vi "PS-OCTA-OCE-autofocus.vi"() -> ()   [LabVIEW 2024] (continued)
                                n349 = call "ORS_Fit_Recalibration_Fringes_Jay.vi"("polynomial order"="poly order", "n Recalibration Fringes"=w812, "polynomial fit algorithm"=T11."LU Decomposition" ("poly fit algo"), "moving average half width"="moving avg win", "interpolation method"=w828, "doPolyFit"="doPolyFit", "Offset"=w791, "Length"=w790) -> ("maxphase"=w795:dbl, "phase"=w797:dbl[], "inverted phase"=w804:dbl[], "rel.phase error"=w807:dbl[])  [unwired: 4 in]
                                n350 = for {
                                tunnel: w823 -> [w839] mode=indexing
                                tunnel: [w838] -> w811 mode=indexing
                                n351 = call-poly <vilib>:"Mean.vi"("X"=w839) -> ("mean"=w838:dbl)  [unwired: 1 out]
                                }
                                n352 = disable-structure shown="Disabled" {
                                disable-tunnel: w807 -> [w831 _]
                                frame Disabled {
                                "Debug: Rel. phase error" <- w831
                                }
                                frame Enabled {
                                }
                                }
                                n353 = Array Size(array=w797) -> (size(s)=w799:i32)
                                n354 = call-poly <vilib>:"Ramp Pattern.vi"("start"=0.0, "end"=1.0, "samples"=w799) -> ("Ramp Pattern"=w796:dbl[])  [unwired: 7 in, 1 out]
                                n355 = call "ORS_linearize_Hilbert.vi"("# zeros added"="# zeros added", "Ch1 Michelson"=w811, "Hilbert in"=w797, "interpolation method"=w824) -> ("Ch1 linearized"=w822:dbl[])  [unwired: 6 in, 1 out]
                                n356 = case shown="True" "DoInterp" {
                                tunnel: w797 -> [_ w837]
                                tunnel: [w832 w837] -> w806
                                tunnel: [w832 w833] -> w805
                                tunnel: w804 -> [_ w834]
                                tunnel: w796 -> [w832 _]
                                frame False {
                                }
                                frame True {
                                n357 = In Range and Coerce(upper limit=1.0, x=w834, lower limit=0.0) -> (coerced(x)=w833:dbl[])  [unwired: 1 out]
                                }
                                }
                                n358 = Bundle By Name("Y"=w822, "dt"=w821) -> (w820:waveform(dbl))  [unwired: 1 in]
                                n359 = call-poly <vilib>:"Extract Single Tone Information.vi"("time signal in"=w820) -> ("detected frequency"=→"detected frequency":dbl)  [unwired: 5 in, 5 out]
                                n360 = Build Array(w806, w805) -> (w802:dbl[][])
                                n361 = Transpose 2D Array(2D array=w802) -> (transposed array=w801:dbl[][])
                              }
                              n362 = case shown="False" "DualCali" {
                                tunnel: w676 -> [w688 w760]
                                tunnel: w674 -> [w687 w759]
                                tunnel: w668 -> [w686 w758]
                                tunnel: w666 -> [w685 w757]
                                tunnel: w665 -> [w684 w756]
                                tunnel: w664 -> [w683 w755]
                                tunnel: [w682 w754] -> w663
                                tunnel: [w679 w753] -> w660
                                tunnel: w661 -> [w679 w753]
                                tunnel: "2ndCali" -> [w681 _]
                                tunnel: w658 -> [w680 _]
                                tunnel: w657 -> [w678 _]
                                frame True {
                                n363 = case shown="True" w686 {
                                tunnel: w688 -> [_ w698]
                                tunnel: [w689 w697] -> w682
                                tunnel: w687 -> [_ w696]
                                tunnel: w685 -> [w689 w694]
                                tunnel: w683 -> [_ w693]
                                tunnel: w684 -> [_ w695]
                                tunnel: w681 -> [_ w692]
                                tunnel: w680 -> [_ w691]
                                tunnel: w678 -> [_ w690]
                                frame False {
                                }
                                frame True {
                                n364 = case shown="True" w692 {
                                tunnel: w698 -> [w701 w710]
                                tunnel: [w702 w709] -> w697
                                tunnel: w696 -> [_ w708]
                                tunnel: w695 -> [_ w707]
                                tunnel: w694 -> [w702 w706]
                                tunnel: w693 -> [_ w705]
                                tunnel: w691 -> [_ w704]
                                tunnel: w690 -> [w699 w703]
                                frame False {
                                n365 = Multiply(x=w701, y=w699) -> (x*y=→"caliphase":dbl[][])
                                }
                                frame True {
                                n366 = stacked-sequence {
                                seq-local: [w713 _] -> [_ w724]
                                tunnel: w710 -> [w722 w730]
                                tunnel: [_ w729] -> w709
                                tunnel: w708 -> [_ w728]
                                tunnel: w707 -> [_ w727]
                                tunnel: w706 -> [_ w726]
                                tunnel: w705 -> [_ w725]
                                tunnel: w704 -> [w712 _]
                                tunnel: w703 -> [w720 _]
                                frame #0 {
                                w717 = 0 ("index (row)")
                                n367 = Multiply(x=w722, y=w720) -> (x*y=w721:dbl[][])
                                n368 = local read "caliphase"() -> (w723:dbl[][])
                                n369 = Subtract(x=w721, y=w723) -> (x-y=w715:dbl[][])
                                n370 = Absolute Value(x=w715) -> (abs(x)=w714:dbl[][])
                                n371 = Index Array(array=w714, index (row)=w717, index (col)=w717) -> (element=w718:dbl)
                                n372 = Subtract(x=w714, y=w718) -> (x-y=w716:dbl[][])
                                n373 = Array Max & Min(array=w716) -> (max value=w719:dbl)  [unwired: 3 out]
                                n374 = Divide(x=w716, y=w719) -> (x/y=w713:dbl[][])
                                n375 = Subtract(x=w713, y=w712) -> (x-y=→"phasedif":dbl[][])
                                }
                                frame #1 {
                                n376 = case shown="False" w727 {
                                tunnel: w730 -> [_ _]
                                tunnel: [w732 w749] -> w729
                                tunnel: w728 -> [w736 w752]
                                tunnel: w726 -> [w734 w748]
                                tunnel: w725 -> [w733 w750]
                                tunnel: w724 -> [w731 w746]
                                frame True {
                                n377 = for {
                                N: 2 -> [_]
                                tunnel: w731 -> [w737]
                                tunnel: w736 -> [w745]
                                tunnel: w733 -> [w743]
                                shift-right: [w741] -> w732
                                shift-left: w734 -> [w740]
                                i -> [w744]
                                n378 = Subtract(x=w743, y=w744) -> (x-y=w738:i32)
                                n379 = Index Array(array=w740, index=w738) -> (element=w742:T13)
                                n380 = Bundle By Name(cluster=w742, "RecalFringePhaseFit"=w737, "RawRecalFringeArray"=w745) -> (w739:T13)
                                n381 = Replace Array Subset(array=w740, new element=w739, index=w738) -> (w741:T8)
                                }
                                }
                                frame False {
                                n382 = Index Array(array=w748, index=w750) -> (element=w751:T13)
                                n383 = Bundle By Name(cluster=w751, "RecalFringePhaseFit"=w746, "RawRecalFringeArray"=w752) -> (w747:T13)
                                n384 = Replace Array Subset(array=w748, new element=w747, index=w750) -> (w749:T8)
                                }
                                }
                                }
                                }
                                }
                                }
                                }
                                }
                                }
                                frame False {
                                n385 = case shown="True" w758 {
                                tunnel: w760 -> [_ w767]
                                tunnel: [w761 w766] -> w754
                                tunnel: w759 -> [_ w765]
                                tunnel: w757 -> [w761 w763]
                                tunnel: w755 -> [_ w762]
                                tunnel: w756 -> [_ w764]
                                frame False {
                                }
                                frame True {
                                n386 = case shown="False" w764 {
                                tunnel: w767 -> [w773 w789]
                                tunnel: [w768 w785] -> w766
                                tunnel: w765 -> [w772 w788]
                                tunnel: w763 -> [w770 w784]
                                tunnel: w762 -> [w769 w786]
                                frame True {
                                n387 = for {
                                N: 2 -> [_]
                                tunnel: w773 -> [w782]
                                tunnel: w772 -> [w781]
                                tunnel: w769 -> [w779]
                                shift-right: [w777] -> w768
                                shift-left: w770 -> [w776]
                                i -> [w780]
                                n388 = Subtract(x=w779, y=w780) -> (x-y=w774:i32)
                                n389 = Index Array(array=w776, index=w774) -> (element=w778:T13)
                                n390 = Bundle By Name(cluster=w778, "RecalFringePhaseFit"=w782, "RawRecalFringeArray"=w781) -> (w775:T13)
                                n391 = Replace Array Subset(array=w776, new element=w775, index=w774) -> (w777:T8)
                                }
                                }
                                frame False {
                                n392 = Index Array(array=w784, index=w786) -> (element=w787:T13)
                                n393 = Bundle By Name(cluster=w787, "RecalFringePhaseFit"=w789, "RawRecalFringeArray"=w788) -> (w783:T13)
                                n394 = Replace Array Subset(array=w784, new element=w783, index=w786) -> (w785:T8)
                                }
                                }
                                }
                                }
                                }
                              }
                            }
                            n395 = Transpose 2D Array(2D array=w651) -> (transposed array=→"Debug: Final phase fit":dbl[][])
                            n396 = Bundle By Name(cluster=w653, "Per Channel Params"=w648) -> (w655:T7)
                          }
                        }
                      }
                      frame #2 {
                        n397 = case shown="\"RecalFringe\", \"RecalFringesMirror\"" w864 {
                          frame "False", Default {
                          }
                          frame "RecalFringe", "RecalFringesMirror" {
                            n398 = Get Date/Time String(want seconds? (F)=TRUE ("Angabe von Sekunden? (F)")) -> (time string=→"Time of last RecalFringes":string)  [unwired: 2 in, 1 out]
                          }
                        }
                        n399 = local write "Acquire Recal Fringes with Mirror"(FALSE ("Capture background")) -> ()
                        n400 = local write "Apply Acq Config"(TRUE ("Apply Acq Config")) -> ()
                        n401 = Build Array (concatenate)(w866, "SaveState") -> (w867:string[])
                      }
                    }
                  }
                }
              }
            }
          }
          frame "Img:Preview" {
            # "Mode/ Tab selector"
            n402 = feedback #2() -> (w871:bool)  [unwired: 1 in]
            n403 = stacked-sequence {
              seq-local: [w913 _] -> [_ w1102]
              seq-local: [w897 _] -> [_ w1082]
              seq-local: [w903 _] -> [_ w1081]
              seq-local: [w912 _] -> [_ w1098]
              seq-local: [w911 _] -> [_ w1096]
              seq-local: [w910 _] -> [_ w1095]
              seq-local: [w909 _] -> [_ w1094]
              seq-local: [w908 _] -> [_ w1093]
              seq-local: [w907 _] -> [_ w1091]
              seq-local: [w906 _] -> [_ w1089]
              seq-local: [w905 _] -> [_ w1087]
              seq-local: [w904 _] -> [_ w1084]
              seq-local: [w896 _] -> [_ w1080]
              seq-local: [w945 _] -> [_ w1090]
              seq-local: [w917 _] -> [_ w1086]
              tunnel: w895 -> [w956 _]
              tunnel: w894 -> [w913 _]
              tunnel: w890 -> [w903 _]
              tunnel: w888 -> [w912 _]
              tunnel: w886 -> [w911 _]
              tunnel: w884 -> [w910 _]
              tunnel: w883 -> [w909 _]
              tunnel: w882 -> [w908 _]
              tunnel: w880 -> [w907 _]
              tunnel: w879 -> [w906 _]
              tunnel: w877 -> [w905 _]
              tunnel: w876 -> [w916 _]
              tunnel: w874 -> [w904 _]
              tunnel: w871 -> [_ _]
              tunnel: [_ w1101] -> w893
              tunnel: [_ w1082] -> w872
              tunnel: [_ w1100] -> w892
              tunnel: [_ w1081] -> w891
              tunnel: [_ w1099] -> w889
              tunnel: [_ w1097] -> w887
              tunnel: [_ w1085] -> w885
              tunnel: [_ w1092] -> w881
              tunnel: [_ w1088] -> w878
              tunnel: [_ w1086] -> w875
              tunnel: [_ w1083] -> w873
              frame #0 {
                # "Store all imaging parameters in the general state cluster"
                n404 = local read "Free running"() -> (w946:bool)
                n405 = Select(t=0, s=w946, f=-1) -> (s? t:f=w902:i32)
                n406 = Empty Array?(array=w916) -> (empty?=w915:bool)
                n407 = case shown="True" "show overlay?" {
                  tunnel: w916 -> [w1056 w1061]
                  tunnel: [w1057 w1063] -> w917
                  tunnel: w915 -> [w1058 w1062]
                  frame False {
                    n408 = case shown="False" w1058 {
                      tunnel: [u8[][] [] w1060] -> w1057
                      tunnel: w1056 -> [_ w1060]
                      frame False {
                      }
                      frame True {
                      }
                    }
                  }
                  frame True {
                    n409 = case shown="True" w1062 {
                      tunnel: [w1064 w1069] -> w1063
                      tunnel: w1061 -> [w1064 _]
                      frame False {
                      }
                      frame True {
                        n410 = Build Path(base path=path "states", name or relative path="overlay image name") -> (appended path=w1071:path)
                        n411 = call <vilib>:"Read PNG File.vi"("path to PNG file"=w1071) -> ("error out"=w1066:errorcluster, "image data"=w1070:T21)  [unwired: 8 in, 1 out]
                        n412 = Unbundle By Name(w1066) -> ("status"=w1068:bool)
                        n413 = call <vilib>:"Unflatten Pixmap.vi"("image data"=w1070) -> ("8-bit pixmap"=w1069:u8[][])  [unwired: 4 in, 6 out]
                        n414 = Not(x=w1068) -> (.not. x?=w1067:bool)
                        n415 = local write "show overlay?"(w1067) -> ()
                      }
                    }
                  }
                }
                n416 = event shown="[0] Timeout" {
                  selector: _ -> [_ _ _ _ _ _ _ _ _ _]
                  dyn-events: _ -> [_ _ _ _ _ _ _ _ _ _]
                  timeout: w902 -> [_ _ _ _ _ _ _ _ _ _]
                  tunnel: [_ _ _ TRUE _ _ _ _ _ _] -> w897
                  tunnel: ["DoPreview" "DoPreview" "DoPreview" "none" "none" "Scan3D" "DoPreview" "DoPreview" "DoPreview" "Do Preview"] -> w896
                  tunnel: "OCE_control" -> [_ _ _ _ _ _ _ w993 _ _]
                  tunnel: "OCT_control" -> [_ _ _ _ _ _ _ _ w1015 _]
                  tunnel: "OCTA_control" -> [_ _ _ _ _ _ w968 _ _ _]
                  tunnel: "Robot_control" -> [_ _ _ _ _ _ _ _ _ w1034]
                  event Timeout {
                    n417 = event-data() -> ()  [unwired: 1 in, 2 out]
                  }
                  event "3D preview": Value Change {
                    n418 = event-data() -> ()  [unwired: 1 in, 6 out]
                    n419 = local write "Apply Config"(TRUE ("Apply Config")) -> ()
                  }
                  event "Apply Acq param": Value Change {
                    n420 = event-data() -> ()  [unwired: 1 in, 6 out]
                    n421 = local write "Apply Config"(TRUE ("Apply Config")) -> ()
                  }
                  event "exit": Mouse Down; "exit": Key Down {
                    n422 = event-data() -> ()  [unwired: 1 in, 5 out]
                  }
                  event "OpModeTab": Value Change {
                    n423 = event-data() -> ()  [unwired: 1 in, 6 out]
                  }
                  event "Start 3D scan": Mouse Down; "Start 3D scan": Key Down; "trigger_scan": Value Change {
                    n424 = event-data() -> ()  [unwired: 1 in, 4 out]
                  }
                  event "OCTA_control": Value Change {
                    n425 = event-data() -> ()  [unwired: 1 in, 6 out]
                    n426 = local read "3D_Galvo_Params"() -> (w969:T4)
                    n427 = case shown="True" w968 {
                      tunnel: [w972 w988] -> w971
                      tunnel: w969 -> [w972 w989]
                      frame False {
                      }
                      frame True {
                        w973 = FALSE
                        n428 = local write "Apply Config"(TRUE) -> ()
                        n429 = local read "3D_Galvo_Params2_OCTA"() -> (w987:T4)
                        n430 = local write "OCT_control"(w973) -> ()
                        n431 = local write "Robot_control"(w973) -> ()
                        n432 = local write "OCE_control"(w973) -> ()
                        n433 = Unbundle By Name(w987) -> ("mode"=w986:i32, "n_lines"=w985:i32, "f_per_pos"=w984:i32, "n_frames"=w983:i32, "X center"=w982:dbl, "X span"=w981:dbl, "Y center"=w980:dbl, "Y span"=w979:dbl, "flyb.lines"=w978:i32, "galvo phase"=w977:i32, "n_dataset"=w976:u32, "flyback fr"=w975:u16)
                        n434 = Bundle By Name(cluster=w989, "mode"=w986, "n_lines"=w985, "f_per_pos"=w984, "n_frames"=w983, "X center"=w982, "X span"=w981, "Y center"=w980, "Y span"=w979, "flyb.lines"=w978, "galvo phase"=w977, "n_dataset"=w976, "flyback fr"=w975) -> (w988:T4)
                      }
                    }
                    n435 = local write "3D_Galvo_Params"(w971) -> ()
                  }
                  event "OCE_control": Value Change {
                    n436 = event-data() -> ()  [unwired: 1 in, 6 out]
                    n437 = local read "3D_Galvo_Params"() -> (w991:T4)
                    n438 = case shown="True" w993 {
                      tunnel: [w994 w1010] -> w992
                      tunnel: w991 -> [w994 w1011]
                      frame False {
                      }
                      frame True {
                        w995 = FALSE
                        n439 = local write "Apply Config"(TRUE) -> ()
                        n440 = local read "3D_Galvo_Params3_OCE"() -> (w997:T4)
                        n441 = local write "OCTA_control"(w995) -> ()
                        n442 = local write "OCT_control"(w995) -> ()
                        n443 = local write "Robot_control"(w995) -> ()
                        n444 = Unbundle By Name(w997) -> ("mode"=w1009:i32, "n_lines"=w1008:i32, "f_per_pos"=w1007:i32, "n_frames"=w1006:i32, "X center"=w1005:dbl, "X span"=w1004:dbl, "Y center"=w1003:dbl, "Y span"=w1002:dbl, "flyb.lines"=w1001:i32, "galvo phase"=w1000:i32, "n_dataset"=w999:u32, "flyback fr"=w998:u16)
                        n445 = Bundle By Name(cluster=w1011, "mode"=w1009, "n_lines"=w1008, "f_per_pos"=w1007, "n_frames"=w1006, "X center"=w1005, "X span"=w1004, "Y center"=w1003, "Y span"=w1002, "flyb.lines"=w1001, "galvo phase"=w1000, "n_dataset"=w999, "flyback fr"=w998) -> (w1010:T4)
                      }
                    }
                    n446 = local write "3D_Galvo_Params"(w992) -> ()
                  }
                  event "OCT_control": Value Change {
                    n447 = event-data() -> ()  [unwired: 1 in, 6 out]
                    n448 = local read "3D_Galvo_Params"() -> (w1014:T4)
                    n449 = case shown="True" w1015 {
                      tunnel: w1014 -> [w1016 w1022]
                      tunnel: [w1016 w1019] -> w1013
                      frame False {
                      }
                      frame True {
                        w1017 = FALSE
                        n450 = local write "Apply Config"(TRUE) -> ()
                        n451 = local read "3D_Galvo_Params4_OCT"() -> (w1021:T4)
                        n452 = local write "OCTA_control"(w1017) -> ()
                        n453 = local write "OCE_control"(w1017) -> ()
                        n454 = local write "Robot_control"(w1017) -> ()
                        n455 = Unbundle By Name(w1021) -> ("mode"=w1033:i32, "n_lines"=w1032:i32, "f_per_pos"=w1031:i32, "n_frames"=w1030:i32, "X center"=w1029:dbl, "X span"=w1028:dbl, "Y center"=w1027:dbl, "Y span"=w1026:dbl, "flyb.lines"=w1025:i32, "galvo phase"=w1024:i32, "n_dataset"=w1023:u32, "flyback fr"=w1020:u16)
                        n456 = Bundle By Name(cluster=w1022, "mode"=w1033, "n_lines"=w1032, "f_per_pos"=w1031, "n_frames"=w1030, "X center"=w1029, "X span"=w1028, "Y center"=w1027, "Y span"=w1026, "flyb.lines"=w1025, "galvo phase"=w1024, "n_dataset"=w1023, "flyback fr"=w1020) -> (w1019:T4)
                      }
                    }
                    n457 = local write "3D_Galvo_Params"(w1013) -> ()
                  }
                  event "Robot_control": Value Change {
                    n458 = event-data() -> ()  [unwired: 1 in, 6 out]
                    n459 = local read "3D_Galvo_Params"() -> (w1037:T4)
                    n460 = case shown="True" w1034 {
                      tunnel: w1037 -> [w1038 w1044]
                      tunnel: [w1038 w1041] -> w1036
                      frame False {
                      }
                      frame True {
                        w1039 = FALSE
                        n461 = local read "3D_Galvo_Params5_Robot"() -> (w1043:T4)
                        n462 = local write "Apply Config"(TRUE) -> ()
                        n463 = local write "OCTA_control"(w1039) -> ()
                        n464 = local write "OCE_control"(w1039) -> ()
                        n465 = local write "OCT_control"(w1039) -> ()
                        n466 = Unbundle By Name(w1043) -> ("mode"=w1055:i32, "n_lines"=w1054:i32, "f_per_pos"=w1053:i32, "n_frames"=w1052:i32, "X center"=w1051:dbl, "X span"=w1050:dbl, "Y center"=w1049:dbl, "Y span"=w1048:dbl, "flyb.lines"=w1047:i32, "galvo phase"=w1046:i32, "n_dataset"=w1045:u32, "flyback fr"=w1042:u16)
                        n467 = Bundle By Name(cluster=w1044, "mode"=w1055, "n_lines"=w1054, "f_per_pos"=w1053, "n_frames"=w1052, "X center"=w1051, "X span"=w1050, "Y center"=w1049, "Y span"=w1048, "flyb.lines"=w1047, "galvo phase"=w1046, "n_dataset"=w1045, "flyback fr"=w1042) -> (w1041:T4)
                      }
                    }
                    n468 = local write "3D_Galvo_Params"(w1036) -> ()
                  }
                }
                n469 = Unbundle By Name(w956) -> ("Per Channel Params"=w958:T8)
                n470 = local read "Dispersion coef"() -> (w943:dbl)
                n471 = local read "cut_level_low"() -> (w954:dbl)
                n472 = local read "cut_level_high"() -> (w953:dbl)
                n473 = local read "crop start"() -> (w955:i32)
                n474 = local read "DVV shift"() -> (w944:i32)
                n475 = for {
                  tunnel: w958 -> [w1079] mode=indexing
                  tunnel: [w1077] -> w957 mode=indexing
                  tunnel: w955 -> [w1078]
                  tunnel: w954 -> [w1076]
                  tunnel: w953 -> [w1075]
                  tunnel: w944 -> [w1074]
                  tunnel: w943 -> [w1073]
                  n476 = Bundle By Name(cluster=w1079, "image crop start"=w1078, "cut_level_low"=w1076, "cut_level_high"=w1075, "DVV_shift"=w1074, "disp_coef"=w1073) -> (w1077:T13)
                }
                n477 = local read "PhaseCompVector"() -> (w928:cdb[])
                n478 = local read "FFT Down Sample"() -> (w924:i32)
                n479 = local read "Dispersion coef"() -> (w927:dbl)
                n480 = local read "cut_level_high"() -> (w923:dbl)
                n481 = local read "IgnoreBadClk"() -> (w920:bool)
                n482 = local read "image height"() -> (w951:i32)
                n483 = local read "DoDispComp"() -> (w929:bool)
                n484 = local read "cut_level_low"() -> (w922:dbl)
                n485 = local read "3D_Galvo_Params"() -> (w949:T4)
                n486 = local read "B scan offset"() -> (w952:dbl)
                n487 = local read "Enable DVV?"() -> (w932:bool)
                n488 = local read "ChannelDisp"() -> (w926:i32)
                n489 = local read "Override Ch."() -> (w934:bool[])
                n490 = local read "Good_Clock"() -> (w919:dbl)
                n491 = local read "Description"() -> (w941:string)
                n492 = local read "Disable Bck"() -> (w930:bool[])
                n493 = local read "ATS_clock 2"() -> (w938:T1)
                n494 = local read "OCT NAME"() -> (w950:string)
                n495 = local read "OCT Zoom"() -> (w925:sgl)
                n496 = local read "Bad_Clock"() -> (w918:dbl)
                n497 = local read "OCT PATH"() -> (w942:path)
                n498 = local read "dual_card"() -> (w940:bool)
                n499 = local read "ATS_clock"() -> (w939:T1)
                n500 = local read "Ch. Select"() -> (w935:bool[])
                n501 = local read "DoInterp"() -> (w933:bool)
                n502 = local read "digi_trig"() -> (w936:bool)
                n503 = local read "Channel"() -> (w921:u32)
                n504 = local read "AO.type"() -> (w931:i32)
                n505 = local read "DES"() -> (w937:bool)
                n506 = Bundle By Name(cluster=w956, "Per Channel Params"=w957, "image height (crop)"=w951, "B scan offset (sps)"=w952, "OCT data dir"=w942, "3d file name"=w950, "Description"=w941, "Galvo params only for file storage"=w949, "do_dual_card"=w940, "ATS_clock"=w939, "ATS_clock 2"=w938, "DES"=w937, "digi_trig"=w936, "Ch. Select"=w935, "Override Ch."=w934, "DoInterp"=w933, "EnableDVV"=w932, "AO.type"=w931, "Disable Bck"=w930, "PhaseCompVector"=w928, "DoDispComp"=w929, "dispcoef"=w927, "ChannelDisp"=w926, "Zoom Factor"=w925, "FFT Down Sample"=w924, "cut_level_high"=w923, "cut_level_low"=w922, "Channel"=w921, "IgnoreBadClk"=w920, "Good_Clock"=w919, "Bad_Clock"=w918) -> (w945:T7)
              }
              frame #1 {
                n507 = case shown="\"DoPreview\"" w1080 {
                  tunnel: w1090 -> [w1175 w1494 w1994]
                  tunnel: w1102 -> [w1201 w1496 w1993]
                  tunnel: [w1175 w1493 w1994] -> w1101
                  tunnel: [w1197 w1495 w1993] -> w1100
                  tunnel: [w1200 _ _] -> w1099
                  tunnel: w1098 -> [w1169 _ _]
                  tunnel: [w1199 _ _] -> w1097
                  tunnel: w1096 -> [w1162 _ _]
                  tunnel: [w1172 _ _] -> w1085
                  tunnel: w1095 -> [w1173 _ _]
                  tunnel: w1094 -> [_ w1492 _]
                  tunnel: w1093 -> [_ w1491 _]
                  tunnel: [w1198 _ _] -> w1092
                  tunnel: w1091 -> [_ _ _]
                  tunnel: w1089 -> [_ _ _]
                  tunnel: [w1161 _ _] -> w1088
                  tunnel: w1087 -> [w1160 _ _]
                  tunnel: w1086 -> [w1184 _ _]
                  tunnel: w1084 -> [w1146 _ _]
                  tunnel: [w1145 _ _] -> w1083
                  frame "DoPreview" {
                    # "frame_width"
                    n508 = stacked-sequence {
                      seq-local: [w1340 _ _ _] -> [_ w1350 _ _]
                      seq-local: [w1343 _ _ _] -> [_ _ _ w1489]
                      seq-local: [w1338 _ _ _] -> [_ w1351 _ _]
                      seq-local: [_ _ w1463 _] -> [_ _ _ w1487]
                      tunnel: w1201 -> [w1341 w1352 _ _]
                      tunnel: [_ w1349 _ _] -> w1197
                      tunnel: [_ _ w1464 _] -> w1172
                      tunnel: [w1338 _ _ _] -> w1200
                      tunnel: [w1340 _ _ _] -> w1199
                      tunnel: [_ _ "B scan offset" _] -> w1198
                      tunnel: [_ _ "ChannelDisp" _] -> w1163
                      tunnel: w1173 -> [_ _ w1465 _]
                      tunnel: [_ _ w1459 _] -> w1167
                      tunnel: [_ _ w1458 _] -> w1166
                      tunnel: [_ _ "Enable SLO" _] -> w1165
                      tunnel: [_ _ w1453 _] -> w1164
                      tunnel: [_ _ w1452 _] -> w1161
                      tunnel: w1160 -> [_ _ w1451 _]
                      frame #0 {
                        n509 = local read "# samples"() -> (w1339:u32)
                        n510 = Tick Count (ms)() -> (millisecond timer value=w1343:u32)
                        n511 = Unbundle By Name(w1341) -> ("n_bit"=w1342:enum16{"8bit", "16bit"})
                        n512 = To Double Precision Float(number=w1339) -> (double precision float=w1338:dbl)
                        "samples/line" <- w1338
                        n513 = local write "n_bit"(w1342) -> ()
                        n514 = Unbundle By Name("3D_Galvo_Params") -> ("n_lines"=w1340:i32)
                        "# lines" <- w1340
                      }
                      frame #1 {
                        n515 = case shown="True" "Apply Config" {
                          tunnel: w1352 -> [w1360 w1411]
                          tunnel: [w1360 w1410] -> w1349
                          tunnel: w1351 -> [_ w1409]
                          tunnel: w1350 -> [_ w1408]
                          tunnel: [w1356 w1379] -> w1347
                          tunnel: [w1363 w1378] -> w1346
                          tunnel: [w1362 w1377] -> w1345
                          tunnel: [w1354 w1374] -> w1344
                          frame False {
                            n516 = Unbundle By Name(w1360) -> ("Galvo"=w1359:T5)
                            n517 = Unbundle By Name(w1359) -> ("params"=w1358:T4)  [unwired: 9 out]
                            n518 = Unbundle By Name(w1358) -> ("mode"=w1361:i32, "f_per_pos"=w1369:i32, "flyback fr"=w1353:u16)  [unwired: 5 out]
                            n519 = Subtract(x=w1361, y=6) -> (x-y=w1367:i32)
                            n520 = Subtract(x=w1369, y=1) -> (x-y=w1370:i32)
                            n521 = Subtract(x=w1361, y=7) -> (x-y=w1368:i32)
                            n522 = Equal To 0?(x=w1367) -> (x = 0?=w1357:bool)
                            n523 = Equal To 0?(x=w1368) -> (x = 0?=w1363:bool)
                            n524 = Equal To 0?(x=w1370) -> (x = 0?=w1372:bool)
                            n525 = And(x=w1357, y=w1372) -> (x .and. y?=w1362:bool)
                            n526 = Not(x=w1372) -> (.not. x?=w1371:bool)
                            n527 = And(x=w1357, y=w1371) -> (x .and. y?=w1356:bool)
                            n528 = Greater?(x=w1353, y=500) -> (0:w1354:bool)
                          }
                          frame True {
                            w1394 = 10178 items=["Finite Samples"=10178, "Continuous Samples"=10123, "Hardware Timed Single Point"=12522] ("SampQuant.SampMode")
                            # "Trigger condition: 1 = no transducer for the preview"
                            n529 = local read "3D_Galvo_Params"() -> (w1403:T4)
                            n530 = local read "3D preview"() -> (w1401:bool)
                            n531 = local read "digi_trig"() -> (w1400:bool)
                            n532 = Unbundle By Name(w1411) -> ("Galvo"=w1404:T5)
                            n533 = Bundle By Name(cluster=w1404, "params"=w1403) -> (w1402:T5)
                            n534 = case shown="False" w1401 {
                              tunnel: [w1416 w1418] -> w1405
                              tunnel: w1402 -> [w1413 w1419]
                              frame True {
                                n535 = local read "XY: Force zero"() -> (w1417:bool)
                                n536 = Bundle By Name(cluster=w1413, "params.force to zero"=w1417, "params.n_dataset"=u32 1, "params.flyback fr"=u16 0, "params.f_per_pos"=1 ("params.frames_per_pos")) -> (w1416:T5)
                              }
                              frame False {
                                n537 = local read "XY: Force zero"() -> (w1423:bool)
                                n538 = Bundle By Name(cluster=w1419, "params.force to zero"=w1423, "params.n_dataset"=u32 1, "params.flyback fr"=u16 0, "params.Y span"=0.0) -> (w1418:T5)
                              }
                            }
                            n539 = call "ORS_GalvoConfig3D_v2.vi"("Galvo"=w1405, "use_digi_trig"=w1400) -> ("Galvo out"=w1392:T5, "error out"=w1406:errorcluster)  [unwired: 16 in]
                            n540 = Unbundle By Name(w1392) -> ()  [unwired: 1 out]
                            n541 = Unbundle By Name(w1392) -> ("params"=w1391:T4)
                            n542 = Unbundle By Name(w1392) -> ("params.Custom trig."=w1398:T22)
                            n543 = Unbundle By Name(w1391) -> ("mode"=w1387:i32, "f_per_pos"=w1384:i32, "flyback fr"=w1376:u16)  [unwired: 5 out]
                            n544 = local read "3D frame"() -> (w1396:i32)
                            n545 = local read "AO.type"() -> (w1399:i32)
                            n546 = Subtract(x=w1387, y=6) -> (x-y=w1389:i32)
                            n547 = Subtract(x=w1387, y=7) -> (x-y=w1386:i32)
                            n548 = Subtract(x=w1384, y=1) -> (x-y=w1383:i32)
                            n549 = Equal To 0?(x=w1386) -> (x = 0?=w1378:bool)
                            n550 = Equal To 0?(x=w1389) -> (x = 0?=w1382:bool)
                            n551 = Equal To 0?(x=w1383) -> (x = 0?=w1380:bool)
                            n552 = call "ORS_GalvoPrepareScan_uw-1kp_Duo.vi"("Galvo"=w1392, "SampQuant.SampMode"=w1394, "3D frame"=w1396, "AO.DataXferMech"=w1399, "Fast Axis/Slow Axis"=TRUE, "use_digi_trig"=w1400, "error in"=w1406, "Trigger condition"=1 ("params.frames_per_pos")) -> ("Galvo out"=w1407:T5)  [unwired: 4 in, 3 out]
                            n553 = And(x=w1382, y=w1380) -> (x .and. y?=w1377:bool)
                            n554 = Bundle By Name(cluster=w1411, "Galvo"=w1407) -> (w1395:T6)
                            n555 = Not(x=w1380) -> (.not. x?=w1381:bool)
                            n556 = Greater?(x=w1376, y=500) -> (0:w1374:bool)
                            n557 = And(x=w1382, y=w1381) -> (x .and. y?=w1379:bool)
                            n558 = Bundle By Name(cluster=w1395, "Galvo.params.Custom trig."=w1398) -> (w1397:T6)
                            n559 = flat-sequence {
                              tunnel: w1397 -> [_]
                              tunnel: w1408 -> [w1425]
                              tunnel: w1409 -> [w1430]
                              tunnel: w1397 -> [w1441]
                              tunnel: [w1440] -> w1410
                              frame #0 {
                                n560 = local read "Laser Trigger"() -> (w1424:bool)
                                n561 = local read "ATSHandle"() -> (w1429:u32[])
                                n562 = local read "Channel"() -> (w1428:u32)
                                n563 = for {
                                tunnel: w1430 -> [w1439]
                                tunnel: w1429 -> [w1438] mode=indexing
                                tunnel: w1428 -> [w1435]
                                tunnel: [w1434] -> w1427
                                tunnel: u32 2147483647 ("Records Count") -> [w1433]
                                tunnel: w1425 -> [w1432]
                                tunnel: w1424 -> [w1431]
                                n564 = call "ORS_AlazarDLLAcq_Prepare.vi"("Lamda Trigger?"=w1431, "Channel"=w1435, "Records Per Buffer"=w1432, "Records Count"=w1433, "Record length"=w1439, "ATSHandle"=w1438) -> ("error out"=w1437:errorcluster, "Samps Per Buffer"=w1434:u32, "ATSHandle_out"=w1436:u32)  [unwired: 3 in]
                                n565 = call "ORS_AlazarDLLAcq_Start.vi"("error in (no error)"=w1437, "ATSHandle"=w1436) -> ()  [unwired: 8 in, 2 out]
                                }
                                "Samps Per Buffer" <- w1427
                              }
                              frame #1 {
                                n566 = Unbundle By Name(w1441) -> ("Galvo"=w1443:T5)
                                n567 = call "ORS_GalvoStartScan.vi"("Galvo"=w1443) -> ("Galvo out"=w1442:T5)  [unwired: 9 in, 1 out]
                                n568 = Bundle By Name(cluster=w1441, "Galvo"=w1442) -> (w1440:T6)
                              }
                            }
                          }
                        }
                        "OCTA_indicator" <- w1347
                        "OCE_indicator" <- w1346
                        "OCT indicator" <- w1345
                        "Robot_indicator" <- w1344
                      }
                      frame #2 {
                        n569 = property on="Raw captured photodiode data" class="WFGraph (strict)"() -> ("CrsrList"=w1460:T9)  [unwired: 2 in, 2 out]
                        n570 = call "ORS_CursorToCropIdx.vi"("index offset"=0, "Cursor List"=w1460) -> ("length"=w1459:i32, "offset"=w1458:i32)  [unwired: 8 in]
                        "a_sca n_offset" <- w1458
                        "a_scan_size" <- w1459
                        n571 = Divide(x=w1459, y=2.0) -> (x/y=→"a_scan_size/2":dbl)
                        n572 = case shown="True" "Freeze" {
                          tunnel: "Freeze" -> [_ w1477]
                          frame False {
                          }
                          frame True {
                            n573 = case shown="True" w1477 {
                              frame True {
                                n574 = local read "ATSHandle"() -> (w1480:u32[])
                                n575 = local write "Apply Config"(FALSE ("Apply Config")) -> ()
                                n576 = Index Array(array=w1480) -> (element=w1479:u32)  [unwired: 1 in]
                                n577 = call "AlazarAbortAsyncRead.vi"("Handle"=w1479) -> ()  [unwired: 1 in, 3 out]
                              }
                              frame False {
                                n578 = local write "Apply Config"(TRUE ("Apply Config")) -> ()
                              }
                            }
                          }
                        }
                        n579 = case shown="False" "Freeze" {
                          tunnel: [w1469 w1471] -> w1468
                          tunnel: [_ w1473] -> w1463
                          tunnel: "ChannelDisp" -> [_ w1472]
                          tunnel: w1465 -> [w1469 _]
                          frame True {
                          }
                          frame False {
                            n580 = local read "Samps Per Buffer"() -> (w1474:u32)
                            n581 = local read "ATSHandle"() -> (w1475:u32[])
                            n582 = call "ORS_AlazarDLLAcq_XferLatestFrame222.vi"("nums"="Interval between displayed OCT frames", "FrameNumToDisplay"=w1472, "SamplesPerBuffer"=w1474, "ATSHandle"=w1475) -> ("Return Code"=w1473:u32, "Buffer"=w1471:u16[])  [unwired: 5 in, 1 out]
                            "Return Code prev" <- w1473
                            n583 = Array Size(array=w1471) -> (size(s)=→"Actual Length":i32)
                          }
                        }
                        n584 = To Long Integer(number=w1468) -> (32bit integer=w1467:i32[])
                        n585 = Subtract(x=w1467, y=32768.0) -> (x-y=w1464:i16[])
                        n586 = Array Size(array=w1464) -> (size(s)=w1453:i32)
                        "input size" <- w1453
                        n587 = Tick Count (ms)() -> (millisecond timer value=w1452:u32)
                        n588 = Subtract(x=w1452, y=w1451) -> (x-y=w1450:u32)
                        n589 = Divide(x=u32 1000, y=w1450) -> (x/y=→"Frame rate":dbl)
                        n590 = Divide(x=w1453, y=w1450) -> (x/y=w1447:dbl)
                        n591 = Multiply(x=0.002, y=w1447) -> (x*y=→"Mb/s transfer rate":dbl)
                      }
                      frame #3 {
                        n592 = Tick Count (ms)() -> (millisecond timer value=w1490:u32)
                        n593 = local read "Freeze"() -> (w1484:bool)
                        n594 = Not(x=w1484) -> (.not. x?=w1483:bool)
                        n595 = Subtract(x=w1490, y=w1489) -> (x-y=→"prev_acq_time":u32)
                        n596 = Not Equal?(x=w1487, y=u32 512) -> (x != y?=w1485:bool)
                        n597 = And(x=w1485, y=w1483) -> (x .and. y?=w1482:bool)
                        n598 = local write "Apply Config"(w1482) -> ()
                      }
                    }
                    n599 = Unbundle By Name(w1175) -> ("Per Channel Params"=w1170:T8)
                    n600 = Divide(x=w1167, y="FFT Down Sample") -> (x/y=w1195:dbl)
                    n601 = Divide(x=w1195, y=2.0) -> (x/y=w1193:dbl)
                    n602 = To Long Integer(number=w1193) -> (32bit integer=w1186:i32)
                    "image height" <- w1186
                    n603 = case shown="False" w1165 {
                      tunnel: [w1232 w1287] -> w1168
                      tunnel: w1166 -> [w1254 _]
                      tunnel: "FFT Down Sample" -> [w1240 _]
                      tunnel: w1167 -> [w1223 _]
                      tunnel: w1170 -> [w1226 w1277]
                      tunnel: w1172 -> [w1242 w1296]
                      tunnel: w1186 -> [w1248 _]
                      tunnel: w1169 -> [w1247 _]
                      tunnel: w1164 -> [w1245 w1295]
                      tunnel: w1162 -> [_ w1286]
                      tunnel: w1163 -> [w1217 _]
                      tunnel: w1162 -> [w1216 _]
                      frame False {
                        n604 = local read "NumCh"() -> (w1231:i32)
                        n605 = Index Array "Index Array"(array=w1226) -> (element=w1225:T13)  [unwired: 1 in]
                        n606 = Unbundle By Name(w1225) -> ("DualBackground"=w1221:i16[], "RecalFringePhaseFit"=w1255:dbl[][])
                        n607 = local read "Enable DVV?"() -> (w1251:bool)
                        n608 = Quotient & Remainder(x=w1245, y=w1231) -> (floor(x/y)=w1230:i32)  [unwired: 1 out]
                        n609 = Index Array "Index Array"(array=w1255) -> (element=w1252:dbl[])  [unwired: 2 in]
                        n610 = Array Size(array=w1252) -> (size(s)=w1222:i32)
                        n611 = Array Subset "Array Subset"(array=w1242, index=w1230, length=w1230) -> (w1250:i16[])
                        n612 = Divide(x=w1230, y=1) -> (x/y=w1243:dbl)
                        n613 = Array Subset "Array Subset"(array=w1242, index=0, length=w1243) -> (w1228:i16[])
                        n614 = Array Subset "Array Subset"(array=w1242, index=w1230, length=w1243) -> (w1241:i16[])
                        n615 = Multiply(x=w1252, y=w1222) -> (x*y=w1236:dbl[])
                        n616 = local read "DoInterp"() -> (w1238:bool)
                        n617 = for {
                          N: w1222 -> [_]
                          tunnel: [w1265] -> w1224 mode=indexing
                          i -> [w1265]
                        }
                        n618 = Select(t=w1222, s=w1238, f=w1223) -> (s? t:f=w1253:i32)
                        n619 = Multiply(x=w1216, y=w1217) -> (x*y=w1215:i32)
                        n620 = case shown="False" w1251 {
                          tunnel: w1247 -> [_ w1272]
                          tunnel: w1254 -> [_ w1268]
                          tunnel: w1223 -> [_ w1269]
                          tunnel: w1215 -> [_ w1274]
                          tunnel: w1250 -> [w1266 w1271]
                          tunnel: [w1266 w1270] -> w1249
                          frame False {
                          }
                          frame True {
                            n621 = local read "Data Valid Vector"() -> (w1267:u32[])
                            n622 = local read "DVV shift"() -> (w1273:i32)
                            n623 = call "ORS_Insight_Reduce_B-scan_Data.vi"("length"=w1269, "offset"=w1268, "Data Valid Vector"=w1267, "spl per line"=w1272, "DVV shift"=w1273, "line Num"=w1274, "Input"=w1271) -> ("Output"=w1270:i16[])  [unwired: 4 in]
                          }
                        }
                        n624 = Bundle(w1247, w1215, "cut_level_high"="cut_level_high", "cut_level_low"="cut_level_low", "offset"=w1254, "length"=w1253, "crop start"="crop start", w1248) -> (w1239:T23)  [unwired: 1 in]
                        n625 = case shown="True" "cal dispcoef" {
                          tunnel: w1249 -> [_ w1264]
                          tunnel: w1221 -> [_ w1263]
                          tunnel: w1215 -> [_ w1262]
                          tunnel: w1247 -> [_ w1261]
                          tunnel: [_ w1258] -> w1227
                          tunnel: w1238 -> [_ w1259]
                          tunnel: w1224 -> [_ w1257]
                          tunnel: w1236 -> [_ w1256]
                          frame False {
                          }
                          frame True {
                            n626 = call "ORS_Phase_Compensation_Fringes.vi"("xi"=w1257, "Do Interp"=w1259, "X"=w1256, "DualBackground"=w1263, "Samples per line"=w1261, "n_lines"=w1262, "Raw Data"=w1264) -> ("dispcoef"=→"Dispersion coef":dbl, "PhaseCompVector"=w1258:cdb[])  [unwired: 3 in]
                          }
                        }
                        "PhaseCompVector" <- w1227
                        n627 = call "ORS_UW_ImgGen.vi"("Disp Comp"="DoDispComp", "Phase Comp Vector"=w1227, "xi"=w1224, "Do Interp"=w1238, "X"=w1236, "imgGen Control"=w1239, "FFT Down Sample"=w1240, "DualBackground"=w1221, "Raw Input"=w1228) -> ("output array"=w1234:u8[])  [unwired: 1 in, 1 out]
                        n628 = call "ORS_UW_ImgGen.vi"("Disp Comp"="DoDispComp", "Phase Comp Vector"=w1227, "xi"=w1224, "Do Interp"=w1238, "X"=w1236, "imgGen Control"=w1239, "FFT Down Sample"=w1240, "DualBackground"=w1221, "Raw Input"=w1241) -> ("output array"=w1235:u8[])  [unwired: 1 in, 1 out]
                        n629 = Insert Into Array(array=w1235, index=0, new element=w1234) -> (w1232:u8[])
                      }
                      frame True {
                        n630 = Index Array(array=w1277) -> (element=w1276:T13)  [unwired: 1 in]
                        n631 = local read "NumCh"() -> (w1294:i32)
                        n632 = Unbundle By Name(w1276) -> ("DualBackground"=w1285:i16[])  [unwired: 2 out]
                        n633 = Quotient & Remainder(x=w1295, y=w1294) -> (floor(x/y)=w1275:i32)  [unwired: 1 out]
                        n634 = for {
                          N: w1286 -> [_]
                          tunnel: w1285 -> [w1297]
                          tunnel: [w1297] -> w1282 mode=concatenating
                        }
                        n635 = Array Subset(array=w1296, index=w1275, length=w1275) -> (w1284:i16[])
                        n636 = To Double Precision Float(number=w1282) -> (double precision float=w1281:dbl[])
                        n637 = Subtract(x=w1284, y=w1281) -> (x-y=w1283:dbl[])
                        n638 = Subtract(x=w1283, y="cut_level_low_SLO") -> (x-y=w1279:dbl[])
                        n639 = Subtract(x="cut_level_high_SLO", y="cut_level_low_SLO") -> (x-y=w1291:dbl)
                        n640 = Absolute Value(x=w1279) -> (abs(x)=w1278:dbl[])
                        n641 = Divide(x=w1278, y=w1291) -> (x/y=w1290:dbl[])
                        n642 = Multiply(x=w1290, y=255.0) -> (x*y=w1280:dbl[])
                        n643 = To Unsigned Byte Integer(number=w1280) -> (unsigned 8bit integer=w1288:u8[])
                        n644 = Decimate 1D Array(w1288) -> (w1287:u8[])  [unwired: 1 out]
                      }
                    }
                    n645 = local read "NumCh"() -> (w1191:i32)
                    n646 = local read "Freeze"() -> (w1155:bool)
                    n647 = Initialize Array "Initialize Array"(u8 255 ("element"), w1186) -> (w1188:u8[])
                    n648 = Not(x=w1155) -> (.not. x?=w1154:bool)
                    n649 = Compound Arithmetic op=MULTIPLY(w1162, w1191, w1163) -> (w1174:i32)
                    n650 = Reshape Array "Reshape Array"(w1168, w1174, w1186) -> (w1190:u8[][])
                    n651 = Array Size(array=w1190) -> (size(s)=w1192:i32[])
                    n652 = Multiply Array Elements(1:w1192) -> (0:w1185:i32)
                    n653 = Replace Array Subset "Replace Array Subset"(array=w1190, new element=w1188, index (row)=w1162) -> (w1187:u8[][])  [unwired: 1 in]
                    n654 = Transpose 2D Array(2D array=w1187) -> (transposed array=w1183:u8[][])
                    n655 = case shown="True" w1154 {
                      tunnel: w1174 -> [_ w1304]
                      tunnel: w1186 -> [_ w1305]
                      tunnel: w1183 -> [_ w1308]
                      tunnel: w1185 -> [_ w1310]
                      tunnel: w1184 -> [_ w1307]
                      tunnel: [w1298 w1303] -> w1145
                      tunnel: w1146 -> [w1298 _]
                      frame False {
                      }
                      frame True {
                        n656 = local read "show overlay?"() -> (w1309:bool)
                        n657 = property on="new picture" class="Pict"("ZoomFactor"="OCT Zoom") -> ()  [unwired: 2 in, 2 out]
                        n658 = call "ORS-ColorTable2ColorMapDataString.vi"("reverse colormap?"="reverse", "Colormap (0 for file/array)"="Colormap") -> ("colors output"=w1300:u32[], "colormap data string"=w1299:string)  [unwired: 8 in]
                        "cmap" <- w1299
                        n659 = case shown="True" w1309 {
                          tunnel: w1308 -> [w1314 w1316]
                          tunnel: [w1314 w1315] -> w1303
                          tunnel: w1307 -> [_ w1317]
                          frame False {
                          }
                          frame True {
                            n660 = Subtract(x=w1316, y=w1317) -> (x-y=w1315:u8[][])
                          }
                        }
                        n661 = case shown="True" "Save?" {
                          tunnel: w1308 -> [_ w1322]
                          tunnel: w1300 -> [_ w1318]
                          frame False {
                          }
                          frame True {
                            n662 = call <vilib>:"Flatten Pixmap.vi"("colors"=w1318, "8-bit pixmap"=w1322) -> ("image data"=w1327:T21)  [unwired: 9 in]
                            n663 = local read "OCT PATH"() -> (w1320:path)
                            n664 = Build Path(base path=w1320, name or relative path="Pic file name") -> (appended path=w1319:path)
                            n665 = call "ORS-PathAddTimestamp.vi"("timestamp?"="Timestamp?", "path"=w1319) -> ("path output"=w1324:path)  [unwired: 9 in]
                            n666 = call "ORS_PathAddNumber_noExt.vi"("format string"="_avg%d", "path"=w1324) -> ("path output"=w1325:path)  [unwired: 9 in]
                            n667 = case shown="False" "JPGorPNG" {
                              tunnel: w1327 -> [w1332 w1336]
                              tunnel: w1325 -> [w1330 w1335]
                              frame False {
                                n668 = call "ORS_PathAddExtension.vi"("new extension"="jpg", "path"=w1330) -> ("appended path"=w1329:path)  [unwired: 9 in]
                                n669 = call <vilib>:"Write JPEG File.vi"("image data"=w1332, "path to JPEG file"=w1329) -> ()  [unwired: 8 in, 2 out]
                              }
                              frame True {
                                n670 = call "ORS_PathAddExtension.vi"("new extension"="png", "path"=w1335) -> ("appended path"=w1334:path)  [unwired: 9 in]
                                n671 = call <vilib>:"Write PNG File.vi"("image data"=w1336, "path to PNG file"=w1334) -> ()  [unwired: 8 in, 2 out]
                              }
                            }
                          }
                        }
                        n672 = Reshape Array "Reshape Array"(w1303, w1310) -> (w1306:u8[])
                        n673 = call "ORS_DrawFlattenedPixmap8.vi"("colormap data string"=w1299, "height"=w1305, "width"=w1304, "image data"=w1306) -> ("new picture"=→"new picture":picture)  [unwired: 5 in]
                      }
                    }
                    n674 = call "robot_state.vi"() -> ("Int from ros"=w1171:i32)  [unwired: 11 in]
                    n675 = local read "scan_flip_state"() -> (w1128:bool)
                    n676 = local read "Robot_control"() -> (w1135:bool)
                    n677 = local read "OCTA_control"() -> (w1124:bool)
                    n678 = local read "OCT_control"() -> (w1134:bool)
                    n679 = local read "OCE_control"() -> (w1133:bool)
                    n680 = local read "3D preview"() -> (w1143:bool)
                    n681 = Not Equal To 0?(x=w1171) -> (x != 0?=w1153:bool)
                    n682 = Not(x="Autofocus") -> (.not. x?=w1114:bool)
                    n683 = call "Is Value Changed.vim"("value"="Autofocus") -> ("changed or first call?"=w1116:bool)
                    n684 = And(x=w1114, y=w1116) -> (x .and. y?=w1113:bool)
                    n685 = Subtract(x="Angle End (deg)", y="Angle Start (deg)") -> (x-y=w1107:dbl)
                    n686 = Not(x=w1153) -> (.not. x?=w1144:bool)
                    n687 = case shown="True" w1113 {
                      frame False {
                      }
                      frame True {
                        n688 = property on="Robot_control" class="Bool (strict)"("Val(Sgnl)"=TRUE) -> ()  [unwired: 2 in, 2 out]
                      }
                    }
                    n689 = Divide(x=w1107, y="Number of points") -> (x/y=→"Angle Increment (deg)":dbl)
                    n690 = Bundle("Robot Vel"="Robot Vel", "Robot Acc"="Robot Acc", "Z-tolerance (mm)"="Z-tolerance (mm)", "Angle tolerance (deg)"="Angle tolerance (deg)", 500, "Radius (mm)"="Radius (mm)", "Angle End (deg)"="Angle End (deg)", "Number of points"="Number of points", w1153, "Z height (pixel)"="Z height (pixel)", "X (mm)"="X (mm)", "Y (mm)"="Y (mm)", "Apply Offset"="Apply Offset", "Angle Start (deg)"="Angle Start (deg)", "N OCT"="N OCT") -> (w1147:T24)  [unwired: 1 in]
                    n691 = case shown="False" "Manual Preview" {
                      tunnel: w1144 -> [w1213 _]
                      frame False {
                        n692 = local write "Freeze"(w1213) -> ()
                      }
                      frame True {
                      }
                    }
                    n693 = Bundle("Autofocus"="Autofocus", "Freedrive"="Freedrive", "Next point"="Next point", "Previous point"="Previous point", "Home"="Home", "Reset"="Reset", "Start Full Protocol"="Start Full Protocol", "3D preview"=w1143, "Robot ON/OFF"="Robot ON/OFF", "Cancel Button"="Cancel Button", "scan_flip_state"=w1128, "Robot_control"=w1135, "OCT_control"=w1134, "OCTA_control"=w1124, "OCE_control"=w1133) -> (w1149:T25)  [unwired: 1 in]
                    n694 = local read "Start 3D scan"() -> (w1121:bool)
                    n695 = Not(x=w1121) -> (.not. x?=w1122:bool)
                    n696 = call "Is Value Changed.vim"("value"=w1128) -> ("changed or first call?"=w1127:bool)
                    n697 = Not(x=w1127) -> (.not. x?=w1126:bool)
                    n698 = call "robot_focus.vi"("Buttons"=w1149, "Parameters"=w1147, "img"=w1145) -> ("Output"=w1150:T26)
                    n699 = Unbundle(w1150) -> ("message"=→"Robot Messages":string, "angle"=→"Current Angle":dbl, "circle_state"=→"Current Point":dbl, "scan_trigger"=w1123:bool, "apply_config"=w1120:bool, "end_state"=w1119:bool, "scan_3d"=w1131:bool, "full_scan"=w1118:bool, "robot_mode"=w1132:bool, "oct_mode"=w1136:bool, "octa_mode"=w1129:bool, "oce_mode"=w1137:bool)
                    n700 = And(x=w1122, y=w1123) -> (x .and. y?=w1125:bool)
                    n701 = And(x=w1125, y=w1126) -> (x .and. y?=w1112:bool)
                    n702 = call "Is Value Changed.vim"("value"=w1118) -> ("changed or first call?"=w1117:bool)
                    n703 = case shown="True" w1112 {
                      frame False {
                      }
                      frame True {
                        n704 = local read "trigger_scan"() -> (w1208:bool)
                        n705 = local write "Start 3D scan"(TRUE) -> ()
                        n706 = Not(x=w1208) -> (.not. x?=w1207:bool)
                        n707 = property on="trigger_scan" class="Bool (strict)"("Val(Sgnl)"=w1207) -> ()  [unwired: 2 in, 2 out]
                      }
                    }
                    n708 = call "Is Value Changed.vim"("value"=w1131) -> ("changed or first call?"=w1139:bool)
                    n709 = case shown="True" w1120 {
                      tunnel: w1120 -> [_ w1211]
                      frame False {
                      }
                      frame True {
                        n710 = property on="Apply Config" class="Bool (strict)"("Val(Sgnl)"=w1211) -> ()  [unwired: 2 in, 2 out]
                      }
                    }
                    n711 = case shown="True" w1119 {
                      frame False {
                      }
                      frame True {
                        n712 = local write "Autofocus"(FALSE) -> ()
                      }
                    }
                    n713 = case shown="True" w1120 {
                      tunnel: w1132 -> [_ w1210]
                      frame False {
                      }
                      frame True {
                        n714 = property on="Robot_control" class="Bool (strict)"("Val(Sgnl)"=w1210) -> ()  [unwired: 2 in, 2 out]
                      }
                    }
                    n715 = case shown="True" w1120 {
                      tunnel: w1136 -> [_ w1204]
                      frame False {
                      }
                      frame True {
                        n716 = property on="OCT_control" class="Bool (strict)"("Val(Sgnl)"=w1204) -> ()  [unwired: 2 in, 2 out]
                      }
                    }
                    n717 = case shown="True" w1120 {
                      tunnel: w1129 -> [_ w1203]
                      frame False {
                      }
                      frame True {
                        n718 = property on="OCTA_control" class="Bool (strict)"("Val(Sgnl)"=w1203) -> ()  [unwired: 2 in, 2 out]
                      }
                    }
                    n719 = case shown="True" w1117 {
                      tunnel: w1118 -> [_ w1209]
                      frame False {
                      }
                      frame True {
                        n720 = property on="Start Full Protocol" class="Bool (strict)"("Val(Sgnl)"=w1209) -> ()  [unwired: 2 in, 2 out]
                      }
                    }
                    n721 = case shown="True" w1120 {
                      tunnel: w1137 -> [_ w1205]
                      frame False {
                      }
                      frame True {
                        n722 = property on="OCE_control" class="Bool (strict)"("Val(Sgnl)"=w1205) -> ()  [unwired: 2 in, 2 out]
                      }
                    }
                    n723 = case shown="True" w1139 {
                      tunnel: w1131 -> [_ w1212]
                      frame False {
                      }
                      frame True {
                        n724 = property on="3D preview" class="Bool (strict)"("Val(Sgnl)"=w1212) -> ()  [unwired: 2 in, 2 out]
                      }
                    }
                    "depth" <- "Z height (pixel)"
                  }
                  frame "Scan3D" {
                    # "BufferSampleArray"
